vi "Pre Launch Init.vi"(11 "DialogBoxSubscribesToDblX in":refnum<class "DialogBoxSubscribesToDblX.lvclass">) -> (0 "error out":errorcluster, 3 "DialogBoxSubscribesToDblX out":refnum<class "DialogBoxSubscribesToDblX.lvclass">)   [LabVIEW 2017, in "DialogBoxSubscribesToDblX.lvclass"]
doc: "(<B>Filename</B>: Actor Framework.lvlib:Actor.lvclass:Pre Launch Init.vi)\n\nDefines behavior that occurs after the Launch Nested Actor method is invoked but before the actor's Actor Core method begins running.\n\nBy default, this method does nothing. A descendant class may override it to define behavior."
uses:
  DialogBoxSubscribesToDblX.lvclass
  C:/Program Files (x86)/National Instruments/LabVIEW 2017/vi.lib/ActorFramework/Actor/Actor.lvclass
  <vilib>/ActorFramework/Actor/Actor.lvclass/Actor.ctl
  <vilib>/ActorFramework/Message Enqueuer/Message Enqueuer.lvclass/Message Enqueuer.ctl
  gpm_packages/@cs/mva-core/Source/IObserver/IObserver Messages/Observe Data Msg/Observe Data Msg.lvclass/Observe Data Msg.ctl
  gpm_packages/@cs/actor-framework-messages/Source/RoundTripMessage/RoundTripMessage.lvclass/RoundTripMessage.ctl
  gpm_packages/@cs/mva-core/Source/IObserver/ActorDataBinding/ActorDataBinding.lvclass/ActorDataBinding.ctl
  gpm_packages/@cs/mva-core/Source/SubscriptionPolicy/ValueChangeSubscription/ValueChangeSubscription.lvclass/ValueChangeSubscription.ctl
  gpm_packages/@cs/mva-core/Source/IMediator/SubscriptionRequest/SubscriptionRequest.lvclass/SubscriptionRequest.ctl
  gpm_packages/@cs/mva-core/Source/IObserver/IObserver Messages/Subscribe Msg/Subscribe Msg.lvclass/Subscribe Msg.ctl
  cff05223-ea57-43ba-ac96-5a028acbdda5.vi
  gpm_packages/@cs/mva-core/Source/IMediator/SubscriptionRequest/Pack Subscription Request.vi
  gpm_packages/@cs/mva-core/Source/SubscriptionPolicy/BasicSubscription/New Basic Subscription.vi
  gpm_packages/@cs/mva-core/Source/SubscriptionPolicy/ValueChangeSubscription/New Value Change Subscription.vi
  gpm_packages/@cs/mva-core/Source/IObserver/ActorDataBinding/New Actor Data Binding Transport.vi
  gpm_packages/@cs/mva-core/Source/IObserver/IObserver Messages/Subscribe Msg/Send Subscribe.vi
  <vilib>/ActorFramework/Actor/Read Self Enqueuer.vi
  gpm_packages/@cs/mva-core/Source/IObserver/IObserver Messages/Observe Data Msg/Write Observe Data Msg Return Info.vi
  <vilib>/ActorFramework/Message Enqueuer/Enqueue.vi
  <vilib>/ActorFramework/Message Enqueuer/Init from Existing Queue.vi
  gpm_packages/@cs/actor-framework-messages/Source/RoundTripMessage/Write Return Address.vi
  gpm_packages/@cs/mva-core/Source/SubscriptionPolicy/ValueChangeSubscription/ValueChangeSubscription.lvclass
  C:/Git/mva-framework/gpm_packages/@cs/mva-core/Source/IMediator/ISubscriptionPolicy/ISubscriptionPolicy.lvclass
  gpm_packages/@cs/mva-core/Source/IObserver/IObserver Messages/Observe Data Msg/Observe Data Msg.lvclass
  C:/Git/mva-framework/gpm_packages/@cs/actor-framework-messages/Source/RoundTripMessage/RoundTripMessage.lvclass
  gpm_packages/@cs/mva-core/Source/IObserver/ActorDataBinding/ActorDataBinding.lvclass
  C:/Git/mva-framework/gpm_packages/@cs/transport/Source/ITransport/ITransport.lvclass
  gpm_packages/@cs/mva-core/Source/IObserver/IObserver Messages/Subscribe Msg/Subscribe Msg.lvclass
  C:/Program Files (x86)/National Instruments/LabVIEW 2017/vi.lib/ActorFramework/Message/Message.lvclass
  <vilib>/ActorFramework/Message Priority Queue/Priority Enqueue.vi
  <vilib>/Utility/error.llb/Error Cluster From Error Code.vi
  gpm_packages/@cs/mva-core/Source/IMediator/ISubscriptionPolicy/Open Subscription Policy.vi
  Source/IDialogBox/IDialogBox/IDialogBox.lvclass
  gpm_packages/@cs/mva-core/Source/IMediator/SubscriptionRequest/SubscriptionRequest.lvclass
  <vilib>/ActorFramework/Message Enqueuer/Message Enqueuer.lvclass
  gpm_packages/@cs/mva-core/Source/SubscriptionPolicy/BasicSubscription/BasicSubscription.lvclass
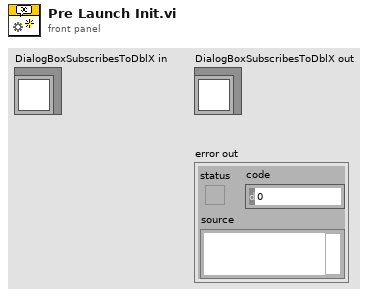
[diagram p1: front panel]
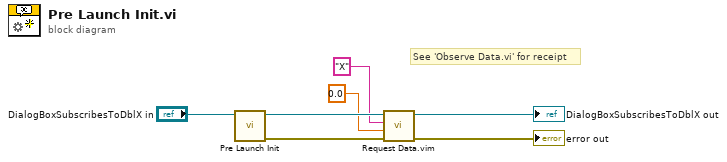
[diagram p0: block diagram]
diagram:
  # "See 'Observe Data.vi' for receipt"
  n1 = call-parent "Pre Launch Init.vi"("IViewable in"="DialogBoxSubscribesToDblX in") -> ("error out"=w7:errorcluster, "IViewable out"=w4:refnum<class "DialogBoxSubscribesToDblX.lvclass">)  [unwired: 9 in]
  n2 = call "Request Data.vim"("error in (no error)"=w7, "Data Type"=0.0, "Datum Name"="X", "IObserver in"=w4) -> ("error out"=→"error out":errorcluster, "IObserver out"=→"DialogBoxSubscribesToDblX out":refnum<class "DialogBoxSubscribesToDblX.lvclass">)  [unwired: 5 in, 1 out]
